vi "Decode Self Test Results.vi"(11 "Status":string) -> (3 "Self-Test Result Message":string)   [LabVIEW 2018, in "XP Power PLS600.lvlib"]
doc: "Decodes the self-test reply into an error message string."
uses:
  XP Power PLS600.lvlib
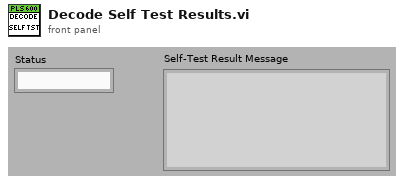
[diagram p1: front panel]
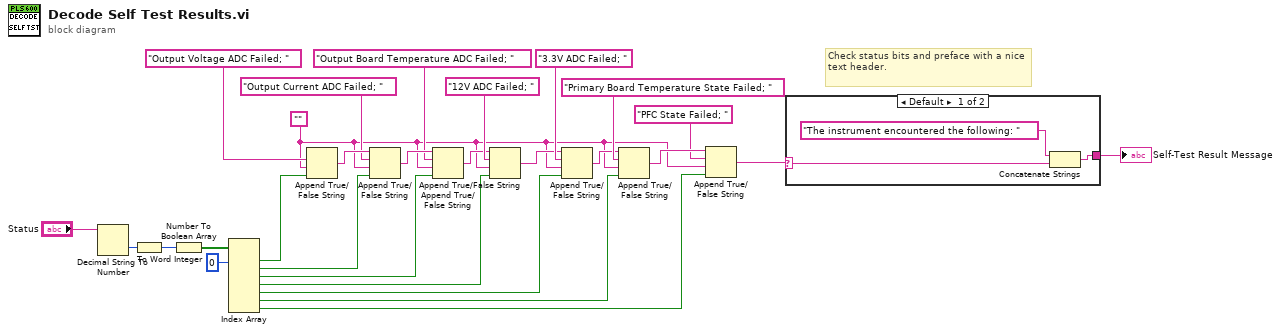
[diagram p0: block diagram]
diagram:
  w8 = ""
  # "Check status bits and preface with a nice text header."
  n1 = Decimal String To Number(string="Status") -> (number=w28:i32)  [unwired: 2 in, 1 out]
  n2 = To Word Integer(number=w28) -> (16bit integer=w2:i16)
  n3 = Number To Boolean Array(number=w2) -> (Boolean array=w19:bool[])
  n4 = Index Array(array=w19, index #1=0 ("index")) -> (element #1=w17:bool, element #2=w16:bool, element #3=w15:bool, element #4=w14:bool, element #5=w5:bool, element #6=w4:bool, element #7=w3:bool)  [unwired: 6 in]
  n5 = Append True/False String(1:w17, 2:w8, 3:"Output Voltage ADC Failed; " ("true string")) -> (0:w26:string)  [unwired: 1 in]
  n6 = Append True/False String(1:w16, 2:w8, 3:"Output Current ADC Failed; " ("true string"), 4:w26) -> (0:w25:string)
  n7 = Append True/False String(1:w15, 2:w8, 3:"Output Board Temperature ADC Failed; " ("true string"), 4:w25) -> (0:w20:string)
  n8 = Append True/False String(1:w14, 2:w8, 3:"12V ADC Failed; " ("true string"), 4:w20) -> (0:w10:string)
  n9 = Append True/False String(1:w5, 2:w8, 3:"3.3V ADC Failed; " ("true string"), 4:w10) -> (0:w11:string)
  n10 = Append True/False String(1:w4, 2:w8, 3:"Primary Board Temperature State Failed; " ("true string"), 4:w11) -> (0:w9:string)
  n11 = Append True/False String(1:w3, 2:w8, 3:"PFC State Failed; " ("true string"), 4:w9) -> (0:w6:string)
  n12 = case shown="Default" w6 {
    selector: w6 -> [w30 w32]
    tunnel: [w29 w32] -> w1
    frame Default {
      n13 = Concatenate Strings("The instrument encountered the following: " ("true string"), w30) -> (w29:string)
    }
    frame "" {
    }
  }
  "Self-Test Result Message" <- w1
